vi "Read Gyro.vi"(8 "error in":errorcluster, 11 "TeleOp Data Cluster in":T1) -> (0 "error out":errorcluster, 3 "TeleOp Data Cluster out":T1)   [LabVIEW 2018]
uses:
  TypeDefs/Teleop Data Cluster.ctl
  TypeDefs/typedef_enum_Refnums.ctl
  <vilib>/Rock Robotics/WPI/ThirdParty/Phoenix-LabVIEW/Pigeon IMU/CTRE_PigeonIMU_GetYPR.vi
  <vilib>/Rock Robotics/Network Tables/NT Write Number.vi
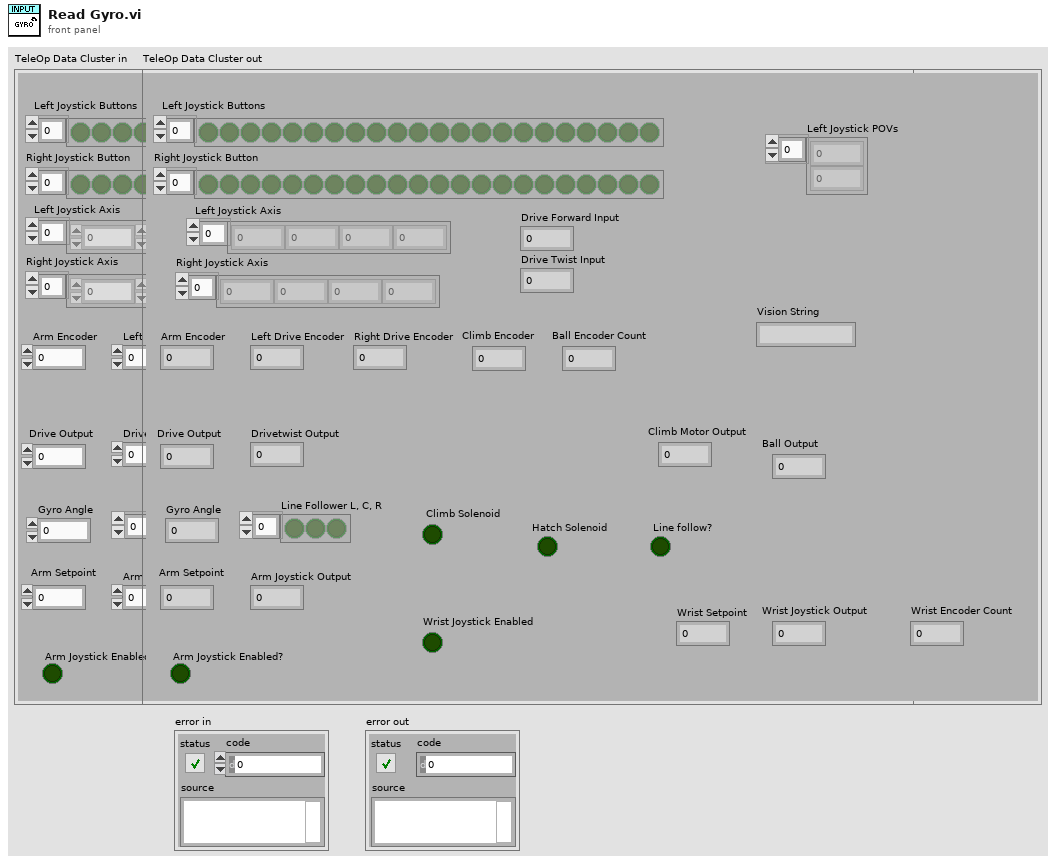
[diagram p1: front panel]
types:
  T1 = typedef "Teleop Data Cluster.ctl" = cluster{"Drive Forward Input ":dbl, "Drive Twist Input":dbl, "Drive Output":dbl, "Drivetwist Output":dbl, "Left Joystick Buttons":bool[], "Left Joystick Axis":dbl[], "Right Joystick Axis":dbl[], "Right Joystick Button":bool[], "Arm Encoder":dbl, "Left Drive Encoder":dbl, "Right Drive Encoder":dbl, "Gyro Angle ":dbl, "Arm Joystick Output  ":dbl, "Line Follower L, C, R ":bool[], "Line follow?":bool, " Climb Solenoid":bool, "Wrist Encoder Count":dbl, "Wrist Joystick Output":dbl, "Ball Encoder Count":dbl, "Ball Output":dbl, "Climb Encoder":dbl, "Climb Motor Output":dbl, " Hatch Solenoid":bool, "Arm Setpoint ":dbl, "Wrist Setpoint ":dbl, "Arm Joystick Enabled?":bool, "Wrist Joystick Enabled":bool, "Vision String":string, "Left Joystick POVs":i16[]}
  T2 = typedef "typedef_enum_Refnums.ctl" = enum16{"Ball_Encoder", "Ball_Motor", "Camera", "Linefollow_3", "Linefollow_2", "Linefollow_1", "Gyro", "Hatch_Solenoid", "Climb_Back_Solenoid", "Arm_Encoder", "Arm_Motor", "Lift_Encoder", "Drive", "Drive_Motor_R", "Drive_Motor_L", "Drive_Encoder_R", "Drive_Encoder_L", "Joy_R", "Joy_L", "Wrist_Motor", "Wrist_Encoder", "Climb Upper Limit", "Climb Lower Limit ", "Climb_Front_Motor"}
  T3 = typedef "CTRE_PigeonIMU_DeviceRef.ctl" = cluster{"DeviceStatus":errorcluster, "Device Number":u8, "Type":T4, "Device ID":u32, "Handle":u64, "UsageFrame":u32, "Library Path":path}
  T4 = typedef "CTRE_PigeonIMU_ConnectionType.ctl" = u32
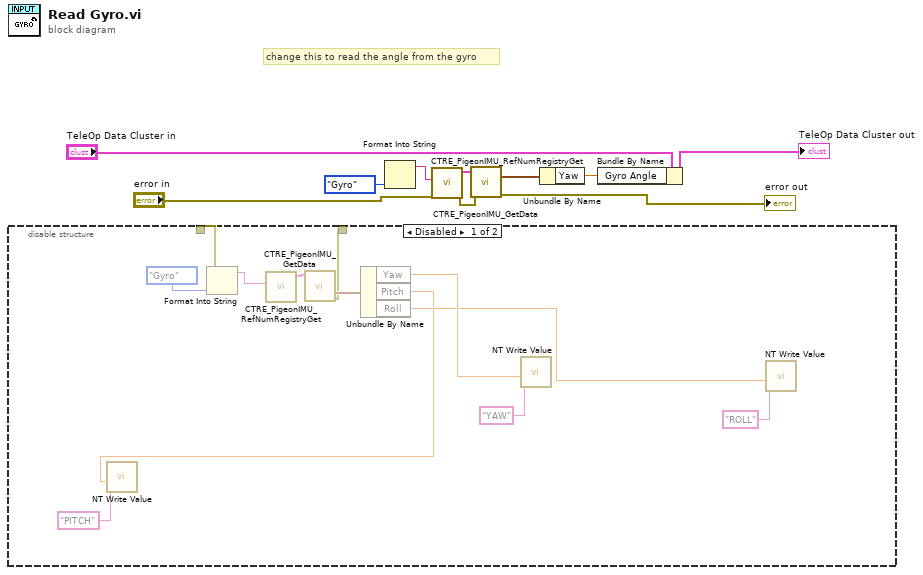
[diagram p0: block diagram]
diagram:
  # "change this to read the angle from the gyro"
  n1 = disable-structure shown="Disabled" {
    disable-tunnel: _ -> [w12 _]
    disable-tunnel: [w11 _] -> _
    frame Disabled {
      n2 = Format Into String(error in=w12, typedef_enum_Refnums."Gyro" ("RefNums")) -> (resulting string=w20:string)  [unwired: 2 in, 1 out]
      n3 = call <vilib>:"CTRE_PigeonIMU_RefNumRegistryGet.vi"("refnum name"=w20) -> ("PigeonIMUDevRef"=w21:T3)  [unwired: 9 in, 1 out]
      n4 = call-poly <vilib>:"CTRE_PigeonIMU_GetData.vi"("PigeonIMUDevRef"=w21) -> ("error out"=w11:errorcluster, "Yaw Pitch Roll"=w19:cluster{"Yaw":dbl, "Pitch":dbl, "Roll":dbl})  [unwired: 8 in, 1 out]
      n5 = Unbundle By Name(w19) -> ("Yaw"=w18:dbl, "Pitch"=w13:dbl, "Roll"=w15:dbl)
      n6 = call-poly <vilib>:"NT Write Value.vi"("Numeric"=w13, "Name"="PITCH") -> ()  [unwired: 9 in, 1 out]
      n7 = call-poly <vilib>:"NT Write Value.vi"("Numeric"=w18, "Name"="YAW") -> ()  [unwired: 9 in, 1 out]
      n8 = call-poly <vilib>:"NT Write Value.vi"("Numeric"=w15, "Name"="ROLL") -> ()  [unwired: 9 in, 1 out]
    }
    frame Enabled {
    }
  }
  n9 = Format Into String(typedef_enum_Refnums."Gyro" ("RefNums")) -> (resulting string=w9:string)  [unwired: 3 in, 1 out]
  n10 = call <vilib>:"CTRE_PigeonIMU_RefNumRegistryGet.vi"("error in (no error)"="error in", "refnum name"=w9) -> ("error out"=w1:errorcluster, "PigeonIMUDevRef"=w2:T3)  [unwired: 8 in]
  n11 = call-poly <vilib>:"CTRE_PigeonIMU_GetData.vi"("error in (no error)"=w1, "PigeonIMUDevRef"=w2) -> ("error out"=→"error out":errorcluster, "Yaw Pitch Roll"=w5:cluster{"Yaw":dbl, "Pitch":dbl, "Roll":dbl})  [unwired: 7 in, 1 out]
  n12 = Unbundle By Name(w5) -> ("Yaw"=w4:dbl)
  n13 = Bundle By Name(cluster="TeleOp Data Cluster in", "Gyro Angle"=w4) -> (→"TeleOp Data Cluster out":T1)
